vi "checkHandshakeRequest.vi"(8 "error in":T1) -> (0 "error out":T1, 3 "HsRequest":bool)   [LabVIEW 2016]
doc: "Verifies whether a manual handshake is expected by the system (HsRequest = True). It can be sent by executing Handshake.vi."
uses:
  Controls/Error_Out.ctl
  Files_ASC500/DLL/ASC500_RemoteControlV27.dll
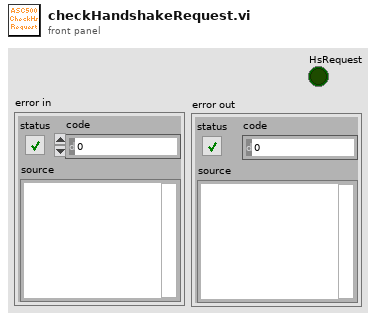
[diagram p1: front panel]
types:
  T1 = typedef "Error_Out.ctl" = errorcluster
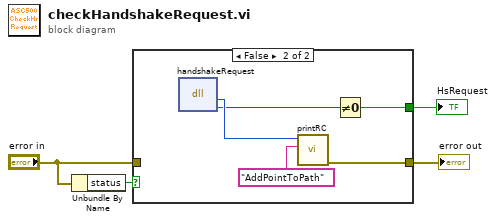
[diagram p0: block diagram]
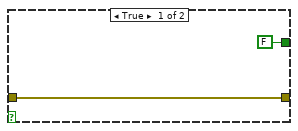
[diagram p2: hidden frame]
diagram:
  n1 = Unbundle By Name("error in") -> ("status"=w2:bool)
  n2 = case shown="False" w2 {
    tunnel: "error in" -> [w6 _]
    tunnel: [w6 w10] -> w4
    tunnel: [FALSE w7] -> w1
    frame True {
    }
    frame False {
      n3 = dll-call lib="G:/SCMOperations/Share/ELE/Produkt Information/ASC500/04 Remote Control/02 development versions/2018Nov06/Files_ASC500/DLL/ASC500_RemoteControlV27.dll" fn="handshakeRequest"() -> ("return type"=w9:i32, "HsReq"=w8:i32)  [unwired: 4 in, 2 out]
      n4 = call "printRC.vi"("additional information"="AddPointToPath", "RC"=w9) -> ("error out"=w10:T1)  [unwired: 9 in]
      n5 = Not Equal To 0?(x=w8) -> (x != 0?=w7:bool)
    }
  }
  "error out" <- w4
  "HsRequest" <- w1
